vi "TestServo.vi"() -> ()   [LabVIEW 2017]
panel:
  in  "Set Servo Position (0 - 180 degrees)":u8(slide)=90 scale=0.0..180.0
  in  "Select Channel":string(combo)="Servo 1"
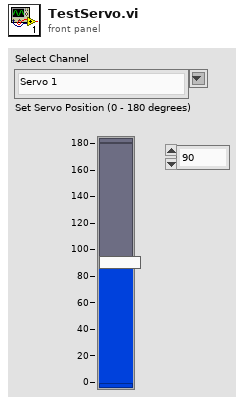
[diagram p1: front panel]
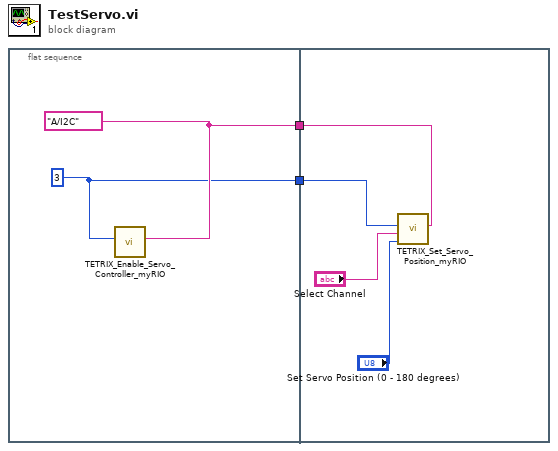
[diagram p0: block diagram]
diagram:
  n1 = flat-sequence {
    tunnel: [w4] -> w2
    tunnel: [w3] -> w1
    tunnel: w2 -> [w8]
    tunnel: w1 -> [w7]
    frame #0 {
      w3 = u8 3 ("Controller ID#  (I2C Address)")
      w4 = tag "A/I2C" ("myRIO MXP Port A/B")
      n2 = call <vilib>:"TETRIX_Enable_Servo_Controller_myRIO.vi"("myRIO MXP Port A/B"=w4, "Controller ID#  (I2C Address)"=w3) -> ()  [unwired: 5 in, 1 out]
    }
    frame #1 {
      n3 = call <vilib>:"TETRIX_Set_Servo_Position_myRIO.vi"("myRIO MXP Port A/B"=w8, "Set Servo Position (0 - 180 degrees)"="Set Servo Position (0 - 180 degrees)", "Select Channel"="Select Channel", "Controller ID#  (I2C Address)"=w7) -> ()  [unwired: 3 in, 1 out]
    }
  }
